vi "Motor Control Enhanced.vi"(0 "PID On":bool) -> (5 "Total (V)":dbl[](array[slide]) scale=-8.0..8.0, 6 "Force (N)":T2(graph)={"M1 ref force"=20.0, "M2 ref force"=20.0, "M1 mes force"=0.47897514031400124, "M2 mes force"=1.2484368104304875})   [LabVIEW 2021]
uses:
  <vilib>/Platform/TimedLoop/XDataNode/timing_clust.ctl
  <vilib>/Platform/TimedLoop/XDataNode/nitl_modes.ctl
  <vilib>/Platform/TimedLoop/XDataNode/wakeup.ctl
  <vilib>/DAQmx/write.llb/DAQmx Write (Digital 1D Bool 1Chan 1Samp).vi
  <vilib>/DAQmx/write.llb/DAQmx Write (Analog 1D DBL NChan 1Samp).vi
  <vilib>/DAQmx/create/channels.llb/DAQmx Create Channel (DO-Digital Output).vi
  <vilib>/DAQmx/create/channels.llb/DAQmx Create Channel (AO-Voltage-Basic).vi
  <vilib>/DAQmx/create/channels.llb/DAQmx Create Channel (AI-Voltage-Basic).vi
  <vilib>/DAQmx/miscellaneous.llb/DAQmx Fill In Error Info.vi
  <vilib>/Platform/TimedLoop/XDataNode/XDataNode.xnode
  <vilib>/Platform/TimedLoop/XDataNode/XDNodeRunTimeDep.lvlib
panel:
  out "Boolean":bool
  in  "Numeric":dbl
  in  "Tab Control":enum32{"PID Gain", "PIN On"}(tab)=enum."PIN On"
  in  "Gains":T1(array[cluster])=[{"proportional gain (Kc)"=0.17, "integral time (Ti, min)"=0.0, "derivative time (Td, min)"=0.0}, {"proportional gain (Kc)"=0.17, "integral time (Ti, min)"=0.0, "derivative time (Td, min)"=0.0}] {"derivative time (Td, min)" format="%.3f"; "integral time (Ti, min)" format="%.3f"; "proportional gain (Kc)" format="%.3f"}
  out "PID (V)":dbl[](array[slide])=[3.31857422614662, 1.0] scale=-8.0..8.0
  out "Trigger":bool
  out "Position (mm)":cluster{"Position":dbl, "ref_x (mm)":dbl}(graph)={"Position"=58.377556358972924, "ref_x (mm)"=0.0}
  in  "Loadcell":bool
  in  "Encoder":bool
  out "In Range?":bool=TRUE
  out "Speed (RPM)":dbl[](array[knob]) scale=-200.0..200.0
  out "time (s)":dbl=642.808
  in  "Set Point":dbl(slide)=19.814241486068113 scale=0.0..40.0
  in  "Motor Enable":bool[](array[boolean])=[FALSE, FALSE]
  in  "stop":bool
  # "FORCE"
  # "TRAJECTORY"
  # "INITIALIZE"
  # "TUNE"
  # "MONITOR"
  # "DEVEL"
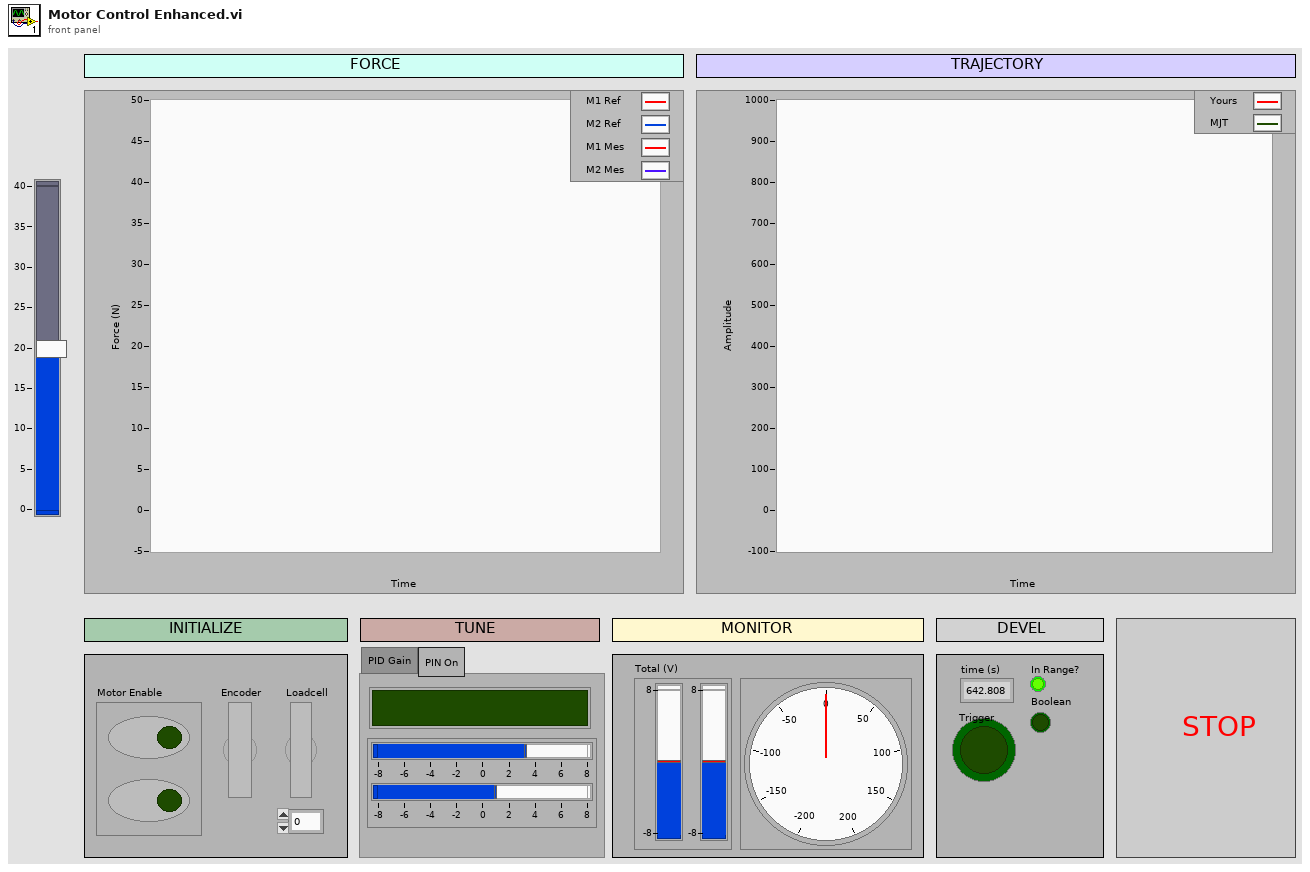
[diagram p1: front panel]
types:
  T1 = cluster{"proportional gain (Kc)":dbl, "integral time (Ti, min)":dbl, "derivative time (Td, min)":dbl}[]
  T2 = cluster{"M1 ref force":dbl, "M2 ref force":dbl, "M1 mes force":dbl, "M2 mes force":dbl}
  T3 = typedef "XDNodeRunTimeDep.lvlib/timing_clust.ctl" = cluster{"Expected End [f-1]":u64, "Actual End [f-1]":u64, "Finished Late? [f-1]":bool, "Expected End [i-1]":u64, "Actual End [i-1]":u64, "Finished Late? [i-1]":bool, "Expected Start [i]":u64, "Actual Start [i]":u64, "Expected Start [f]":u64, "Actual Start [f]":u64, "Source Name":string, "Structure Name":string, "Period":i64, "Deadline":i64, "Offset":i64, "Start":i64, "Priority":i32, "Timeout":i32, "Mode":T4, "Wakeup Reason":T5, "Error":errorcluster, "Source Type":string, "Secondary Source Type":string, "Global End Time":u64, "Global Start Time":u64, "Frame Duration":u64, "Iteration Duration":u64, "Assigned CPU":i32, "I/O Scan Engine Mode":u32}
  T4 = typedef "XDNodeRunTimeDep.lvlib/nitl_modes.ctl" = enum32{"No Change", "Process missed periods, maintain original phase", "Discard missed periods, maintain original phase", "Process missed periods, ignore original phase", "Discard missed periods, ignore original phase"}
  T5 = typedef "XDNodeRunTimeDep.lvlib/wakeup.ctl" = enum32{"Normal", "Aborted", "Asynchronous wakeup", "Timing source error", "Timed loop error", "Timeout"}
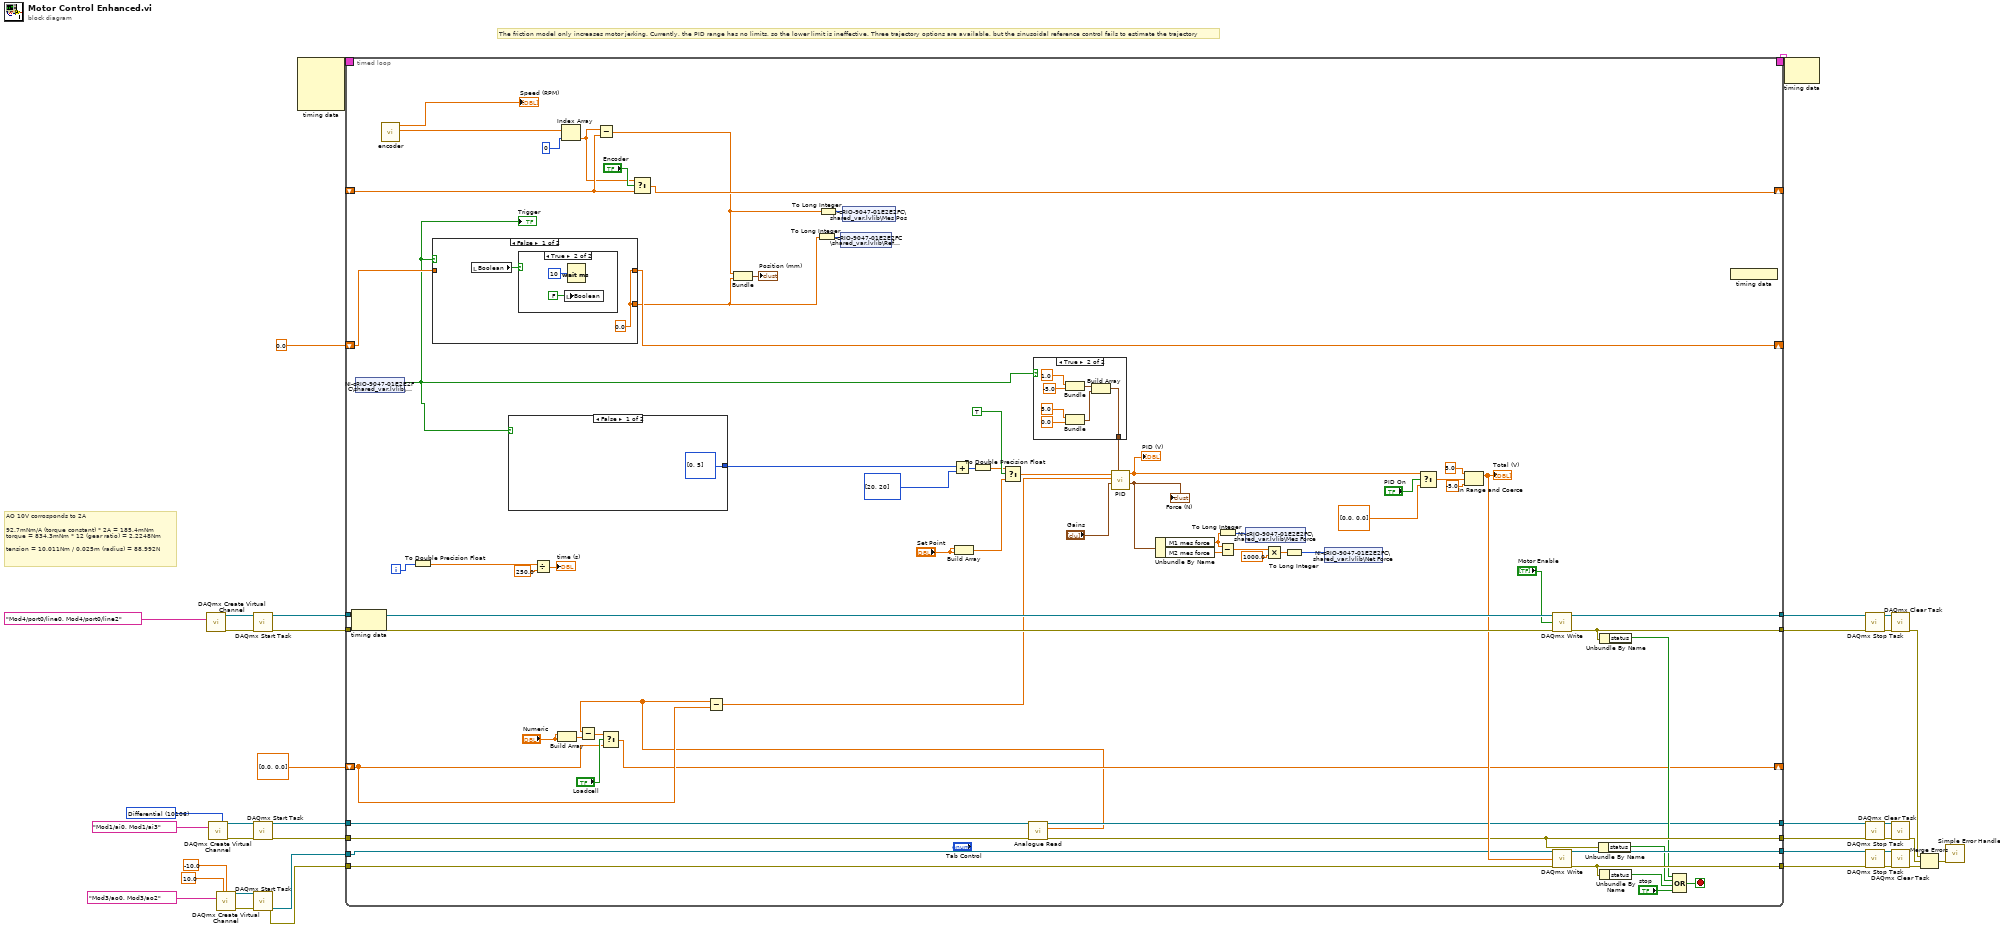
[diagram p0: block diagram]
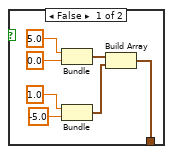
[diagram p2: hidden frame]
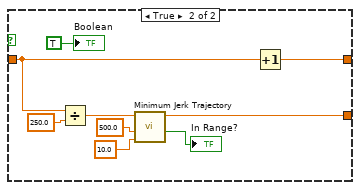
[diagram p4: hidden frame]
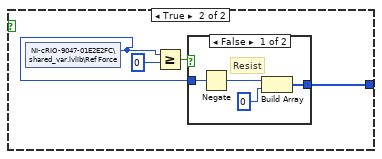
[diagram p5: hidden frame]
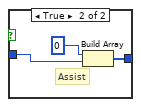
[diagram p6: hidden frame]
diagram:
  w3 = 10106 items=["Default"=-1, "RSE"=10083, "NRSE"=10078, "Differential"=10106, "Pseudodifferential"=12529] ("input terminal configuration")
  # "The friction model only increases motor jerking. Currently, the PID range has no limits, so the lower limit is ineffective. Three trajectory options are available, but the sinusoidal reference control fails to estimate the trajectory"
  # "AO 10V corrosponds to 2A\n\n92.7mNm/A (torque constant) * 2A = 185.4mNm\ntorque = 834.3mNm * 12 (gear ratio) = 2.2248Nm\n\ntension = 10.011Nm / 0.025m (radius) = 88.992N"
  n1 = call-poly <vilib>:"DAQmx Create Virtual Channel.vi"("lines"=tag "Mod4/port0/line0, Mod4/port0/line2") -> ("task out"=w30:refnum<k21>, "error out"=w29:errorcluster)  [unwired: 13 in]
  n2 = call-poly <vilib>:"DAQmx Create Virtual Channel.vi"("input terminal configuration"=w3, "physical channels"=tag "Mod1/ai0, Mod1/ai3") -> ("task out"=w20:refnum<k21>, "error out"=w21:errorcluster)  [unwired: 12 in]
  n3 = call-poly <vilib>:"DAQmx Create Virtual Channel.vi"("maximum value"=10.0 ("AO max"), "minimum value"=-10.0 ("AO min"), "physical channels"=tag "Mod3/ao0, Mod3/ao2" ("Physical Channel(s)")) -> ("task out"=w14:refnum<k21>, "error out"=w13:errorcluster)  [unwired: 11 in]
  n4 = call <vilib>:"DAQmx Start Task.vi"("task/channels in"=w30, "error in"=w29) -> ("task out"=w27:refnum<k21>, "error out"=w26:errorcluster)  [unwired: 12 in]
  n5 = call <vilib>:"DAQmx Start Task.vi"("task/channels in"=w20, "error in"=w21) -> ("task out"=w18:refnum<k21>, "error out"=w17:errorcluster)  [unwired: 12 in]
  n6 = call <vilib>:"DAQmx Start Task.vi"("task/channels in"=w14, "error in"=w13) -> ("task out"=w32:refnum<k21>, "error out"=w31:errorcluster)  [unwired: 12 in]
  n7 = node-c288() -> (w34:T3)  [unwired: 4 in]
  n8 = timed-loop {
    tunnel: [w108] -> w38
    tunnel: [w107] -> w37
    tunnel: [w65] -> w36
    tunnel: [w94] -> w35
    tunnel: w18 -> [w105]
    timing: w34 -> [_]
    timing-out: [_] -> w33
    tunnel: w17 -> [w104]
    tunnel: w32 -> [w64]
    tunnel: w31 -> [w106]
    tunnel: w27 -> [w103]
    tunnel: w26 -> [w102]
    tunnel: [w101] -> w23
    tunnel: [w95] -> w22
    shift-right: [w76] -> _
    shift-left: 0.0 ("total time") -> [w77]
    shift-right: [w71] -> _
    shift-left: _ -> [w69]
    shift-right: [w50] -> _
    shift-left: dbl[] [0.0, 0.0] ("measured force") -> [w51]
    i -> [w82]
    stop <- w90 stop-if-true
    n9 = node-c288() -> ()  [unwired: 1 in, 1 out]
    n10 = shared-variable "NI-cRIO-9047-01E2E2FC\\shared_var.lvlib\\Trigger"() -> (w43:bool)  [unwired: 1 in, 1 out]
    "Trigger" <- w43
    n11 = call "encoder.vi"() -> ("Mes Pos (mm)"=w74:dbl[], "RPM"=→"Speed (RPM)":dbl[])  [unwired: 10 in]
    n12 = To Double Precision Float(number=w82) -> (double precision float=w81:dbl)
    n13 = case shown="False" w43 {
      tunnel: w77 -> [_ w131]
      tunnel: [w126 w134] -> w76
      tunnel: [w126 w130] -> w61
      frame False {
        w126 = 0.0
        n14 = local read "Boolean"() -> (w125:bool)
        n15 = case shown="True" w125 {
          frame False {
          }
          frame True {
            n16 = local write "Boolean"(FALSE ("Boolean")) -> ()
            n17 = Wait (ms)(milliseconds to wait=u32 10) -> ()  [unwired: 1 out]
          }
        }
      }
      frame True {
        n18 = Divide(x=w131, y=250.0) -> (x/y=w132:dbl)
        n19 = call "Minimum Jerk Trajectory.vi"("total time"=10.0, "total length"=500.0, "t (sec)"=w132) -> ("In Range?"=→"In Range?":bool, "ref_x (mm)"=w130:dbl)  [unwired: 7 in]
        n20 = Increment(x=w131) -> (x+1=w134:dbl)
        "Boolean" <- TRUE ("Boolean")
      }
    }
    n21 = case shown="False" w43 {
      tunnel: [i32[] [0, 5] w142] -> w67
      frame False {
      }
      frame True {
        n22 = shared-variable "NI-cRIO-9047-01E2E2FC\\shared_var.lvlib\\Ref Force"() -> (w141:i32)  [unwired: 1 in, 1 out]
        n23 = Greater Or Equal?(x=w141, y=0) -> (x >= y?=w139:bool)
        n24 = case shown="False" w139 {
          tunnel: w141 -> [w145 w148]
          tunnel: [w146 w149] -> w142
          frame False {
            # "Resist"
            n25 = Negate(x=w145) -> (-x=w143:i32)
            n26 = Build Array(w143, 0 ("element")) -> (w146:i32[])
          }
          frame True {
            # "Assist"
            n27 = Build Array(0 ("element"), w148) -> (w149:i32[])
          }
        }
      }
    }
    n28 = Divide(x=w81, y=250.0) -> (x/y=→"time (s)":dbl)
    n29 = Build Array("Numeric", "Numeric") -> (w39:dbl[])
    n30 = Index Array(array=w74, index=0) -> (element=w68:dbl)
    n31 = Subtract(x=w68, y=w69) -> (x-y=w60:dbl)
    n32 = Select(t=w68, s="Encoder", f=w69) -> (s? t:f=w71:dbl)
    n33 = Bundle(w60, "ref_x (mm)"=w61) -> (→"Position (mm)":cluster{dbl, "ref_x (mm)":dbl})  [unwired: 1 in]
    n34 = To Long Integer(number=w61) -> (32bit integer=w46:i32)
    n35 = To Long Integer(number=w60) -> (32bit integer=w45:i32)
    n36 = shared-variable "NI-cRIO-9047-01E2E2FC\\shared_var.lvlib\\Ref Pos"(w46) -> ()  [unwired: 1 in, 1 out]
    n37 = shared-variable "NI-cRIO-9047-01E2E2FC\\shared_var.lvlib\\Mes Pos"(w45) -> ()  [unwired: 1 in, 1 out]
    n38 = Add(x=w67, y=i32[] [20, 20] ("x")) -> (x+y=w63:i32[])
    n39 = Build Array("Set Point", "Set Point") -> (w84:dbl[])
    n40 = To Double Precision Float(number=w63) -> (double precision float=w62:dbl[])
    n41 = Select(t=w62, s=TRUE, f=w84) -> (s? t:f=w57:dbl[])
    n42 = call "Analogue Read.vi"("error in"=w104, "task/channels in"=w105) -> ("error out"=w94:errorcluster, "measured force"=w48:dbl[], "task out"=w65:refnum<k21>)  [unwired: 6 in, 1 out]
    n43 = Subtract(x=w48, y=w39) -> (x-y=w47:dbl[])
    n44 = Select(t=w47, s="Loadcell", f=w51) -> (s? t:f=w50:dbl[])
    n45 = Subtract(x=w48, y=w51) -> (x-y=w49:dbl[])
    n46 = case shown="True" w43 {
      tunnel: [w111 w118] -> w53
      frame False {
        n47 = Bundle(5.0, 0.0) -> (w117:cluster{dbl, dbl})  [unwired: 1 in]
        n48 = Bundle(1.0, -5.0) -> (w116:cluster{dbl, dbl})  [unwired: 1 in]
        n49 = Build Array(w117, w116) -> (w111:cluster{dbl, dbl}[])
      }
      frame True {
        n50 = Bundle(1.0, -5.0) -> (w119:cluster{dbl, dbl})  [unwired: 1 in]
        n51 = Bundle(5.0, 0.0) -> (w120:cluster{dbl, dbl})  [unwired: 1 in]
        n52 = Build Array(w119, w120) -> (w118:cluster{dbl, dbl}[])
      }
    }
    n53 = call "PID.vi"("output range"=w53, "PID gains"="Gains", "mes force"=w49, "ref force"=w57) -> ("output cluster"=w41:T2, "PID output"=w88:dbl[])  [unwired: 6 in]
    "Force (N)" <- w41
    "PID (V)" <- w88
    n54 = Unbundle By Name(w41) -> ("M1 mes force"=w54:dbl, "M2 mes force"=w55:dbl)
    n55 = To Long Integer(number=w54) -> (32bit integer=w56:i32)
    n56 = Subtract(x=w54, y=w55) -> (x-y=w59:dbl)
    n57 = shared-variable "NI-cRIO-9047-01E2E2FC\\shared_var.lvlib\\Mes Force"(w56) -> ()  [unwired: 1 in, 1 out]
    n58 = Multiply(x=w59, y=1000.0) -> (x*y=w42:dbl)
    n59 = To Long Integer(number=w42) -> (32bit integer=w44:i32)
    n60 = shared-variable "NI-cRIO-9047-01E2E2FC\\shared_var.lvlib\\Net Force"(w44) -> ()  [unwired: 1 in, 1 out]
    n61 = Select(t=w88, s="PID On", f=dbl[] [0.0, 0.0]) -> (s? t:f=w86:dbl[])
    n62 = In Range and Coerce(upper limit=5.0, x=w86, lower limit=-5.0) -> (coerced(x)=w96:dbl[])  [unwired: 1 out]
    "Total (V)" <- w96
    n63 = call-poly <vilib>:"DAQmx Write.vi"("task/channels in"=w103, "data"="Motor Enable", "error in"=w102) -> ("task out"=w101:refnum<k21>, "error out"=w95:errorcluster)  [unwired: 10 in, 1 out]
    n64 = call-poly <vilib>:"DAQmx Write.vi"("task/channels in"=w64, "data"=w96, "error in"=w106) -> ("task out"=w108:refnum<k21>, "error out"=w107:errorcluster)  [unwired: 10 in, 1 out]
    n65 = Unbundle By Name(w94) -> ("status"=w92:bool)
    n66 = Unbundle By Name(w95) -> ("status"=w91:bool)
    n67 = Unbundle By Name(w107) -> ("status"=w93:bool)
    n68 = Compound Arithmetic op=OR(w91, w92, w93, "stop") -> (w90:bool)
    n69 = node-c288() -> ()  [unwired: 1 out]
  }
  n70 = node-c288(w33) -> ()  [unwired: 1 out]
  n71 = call <vilib>:"DAQmx Stop Task.vi"("task/channels in"=w23, "error in"=w22) -> ("task out"=w25:refnum<k21>, "error out"=w24:errorcluster)  [unwired: 12 in]
  n72 = call <vilib>:"DAQmx Stop Task.vi"("task/channels in"=w36, "error in"=w35) -> ("task out"=w9:refnum<k21>, "error out"=w8:errorcluster)  [unwired: 12 in]
  n73 = call <vilib>:"DAQmx Stop Task.vi"("task/channels in"=w38, "error in"=w37) -> ("task out"=w11:refnum<k21>, "error out"=w10:errorcluster)  [unwired: 12 in]
  n74 = call <vilib>:"DAQmx Clear Task.vi"("task in"=w25, "error in"=w24) -> ("error out"=w4:errorcluster)  [unwired: 13 in]
  n75 = call <vilib>:"DAQmx Clear Task.vi"("task in"=w9, "error in"=w8) -> ("error out"=w5:errorcluster)  [unwired: 13 in]
  n76 = call <vilib>:"DAQmx Clear Task.vi"("task in"=w11, "error in"=w10) -> ("error out"=w6:errorcluster)  [unwired: 13 in]
  n77 = Merge Errors(w4, w5, w6) -> (w7:errorcluster)
  n78 = call <vilib>:"Simple Error Handler.vi"("error in (no error)"=w7) -> ()  [unwired: 4 in, 5 out]
